vi "Field_Display_Main_Selector.vi"() -> ()   [LabVIEW 2019]
doc: "This WebSockets API example VI acts as a server for an incoming websockets connection. Receives/sends string data to the connected client."
uses:
  <vilib>/Rock Robotics/WPI/ThirdParty/JAS_Junk/TrajLib/TypeDef/FieldDisp_ElementPicture.ctl
  <vilib>/Rock Robotics/WPI/ThirdParty/JAS_Junk/TrajLib/TypeDef/POSE2D.ctl
  <vilib>/Rock Robotics/WPI/ThirdParty/JAS_Junk/TrajLib/TypeDef/TRANSLATION2D.ctl
  <vilib>/Rock Robotics/WPI/ThirdParty/JAS_Junk/TrajLib/TypeDef/ROTATION2D.ctl
  <vilib>/Rock Robotics/WPI/ThirdParty/JAS_Junk/TrajLib/Trajectory_Library.lvlib
panel:
  in  "Robot Pose SI":T1={"TRANSLATION"={"X"=1.0, "Y"=1.0}, "ROTATION"={"VALUE"=0.0, "COS"=1.0, "SIN"=0.0}} {"ROTATION"."SIN" format="%13.4f"; "ROTATION"."COS" format="%13.4f"; "ROTATION"."VALUE" format="%13.4f"; "TRANSLATION"."Y" format="%14.3f"; "TRANSLATION"."X" format="%14.3f"}
  out "ROBOT":T4
  out "Field Picture":picture
  in  "Field Selector":string(combo)
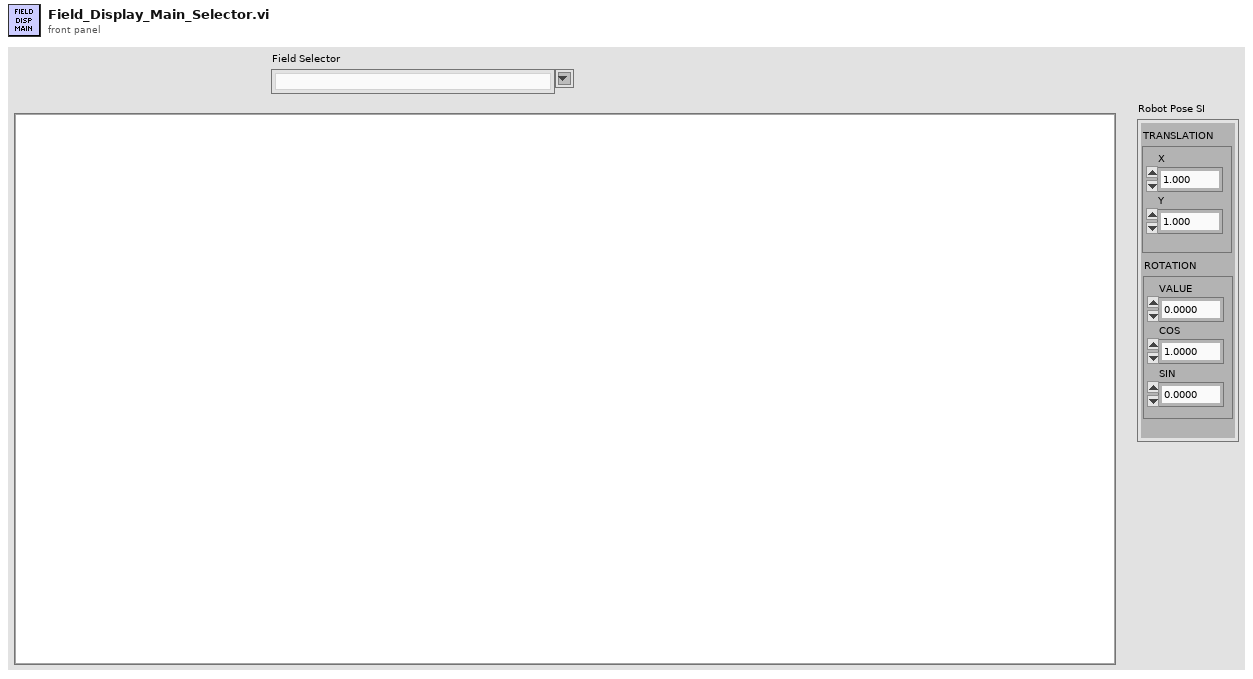
[diagram p1: front panel]
types:
  T1 = typedef "Trajectory_Library.lvlib/POSE2D.ctl" = cluster{"TRANSLATION":T2, "ROTATION":T3}
  T2 = typedef "Trajectory_Library.lvlib/TRANSLATION2D.ctl" = cluster{"X":dbl, "Y":dbl}
  T3 = typedef "Trajectory_Library.lvlib/ROTATION2D.ctl" = cluster{"VALUE":dbl, "COS":dbl, "SIN":dbl}
  T4 = typedef "Trajectory_Library.lvlib/FieldDisp_ElementPicture.ctl" = picture
  T5 = typedef "Trajectory_Library.lvlib/FieldDisp_FieldElement.ctl" = cluster{"ONE-8-bit pixmap":u8[][], "Two-Array":cdb[][], "Three-Numeric":i32, "Four-Numeric":i32, "Five-Numeric":cdb, "Six-colors":u32[], "Seven-new element/subarray":u32, "Left Poxel":dbl, "Top Pixel":dbl, "Width Pix/Ft":dbl, "Height Pix/Ft":dbl, "Element Picture Ref":refnum<vi>}
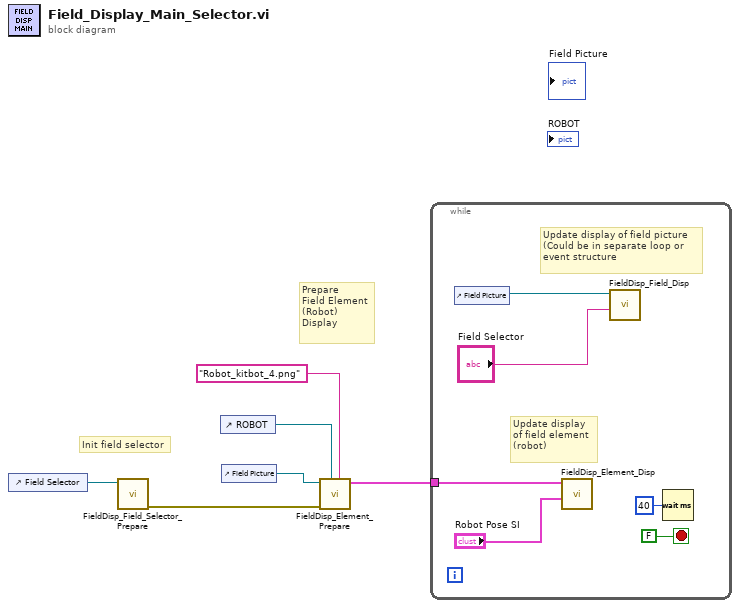
[diagram p0: block diagram]
diagram:
  # "Prepare\nField Element\n(Robot)\nDisplay"
  # "Init field selector"
  n1 = control-ref of="Field Selector"() -> (w6:refnum<vi>)
  n2 = call <vilib>:"FieldDisp_Field_Selector_Prepare.vi"("ComboBox Ref"=w6) -> ("error out"=w5:errorcluster)  [unwired: 9 in, 1 out]
  n3 = control-ref of="ROBOT"() -> (w3:refnum<vi>)
  n4 = control-ref of="Field Picture"() -> (w4:refnum<vi>)
  n5 = call <vilib>:"FieldDisp_Element_Prepare.vi"("Element File Name"="Robot_kitbot_4.png" ("Picture FIle Name"), "Element Picture Ref"=w3, "error in (no error)"=w5, "Field Picture Ref"=w4) -> ("Field Element Info"=w1:T5)  [unwired: 6 in, 1 out]
  n6 = while {
    tunnel: w1 -> [w9]
    stop <- FALSE stop-if-true
    # "Update display of field picture\n(Could be in separate loop or\nevent structure"
    # "Update display\nof field element\n(robot)"
    n7 = control-ref of="Field Picture"() -> (w10:refnum<vi>)
    n8 = call <vilib>:"FieldDisp_Element_Disp.vi"("Element Pose"="Robot Pose SI", "Element Info"=w9) -> ()  [unwired: 10 in]
    n9 = call <vilib>:"FieldDisp_Field_Disp.vi"("Field Selector"="Field Selector", "Picture in"=w10) -> ()  [unwired: 9 in, 1 out]
    n10 = Wait (ms)(milliseconds to wait=u32 40) -> ()  [unwired: 1 out]
  }
